vi "Complex Inverse Matrix.vi"(2 "matrix type":T1, 3 "Input Matrix":T2) -> (0 "error":i32, 1 "Inverse Matrix":T2)   [LabVIEW 2014, in "NI_AALBase.lvlib"]
doc: "Finds <B>Inverse Matrix</B>, if it exists, of <B>Input Matrix</B>. Wire data to the <B>Input Matrix</B> input to determine the polymorphic instance to use or manually select the instance."
uses:
  NI_AALBase.lvlib
  ComplexMatrix.ctl
  Matrix Type of Inverse Matrix.ctl
  NI_Matrix.lvlib
panel:
  # "Complex Inverse Matrix"
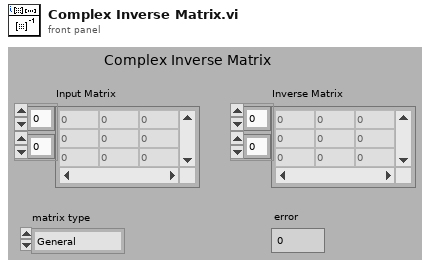
[diagram p1: front panel]
types:
  T1 = typedef "NI_AALBase.lvlib/Matrix Type of Inverse Matrix.ctl" = enum32{"General", "Positive Definite", "Lower Triangular", "Upper Triangular"}
  T2 = typedef "NI_Matrix.lvlib/ComplexMatrix.ctl" = cdb[][]
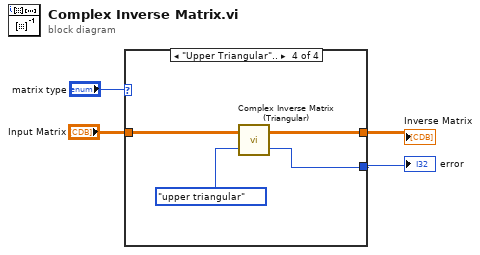
[diagram p0: block diagram]
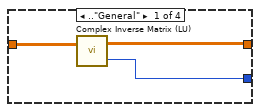
[diagram p2: hidden frame]
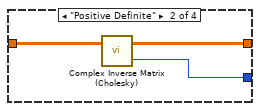
[diagram p3: hidden frame]
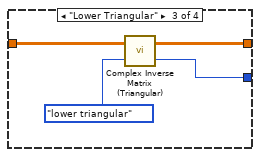
[diagram p4: hidden frame]
diagram:
  n1 = case shown="\"Upper Triangular\".." "matrix type" {
    tunnel: [w5 w9 w13 w17] -> w4
    tunnel: [w7 w10 w14 w18] -> w1
    tunnel: "Input Matrix" -> [w6 w8 w12 w16]
    frame .."General" {
      n2 = call "Complex Inverse Matrix (LU).vi"("A"=w6) -> ("error"=w5:i32, "Inverse Matrix"=w7:T2)  [unwired: 1 in]
    }
    frame "Positive Definite" {
      n3 = call "Complex Inverse Matrix (Cholesky).vi"("Input Matrix"=w8) -> ("error"=w9:i32, "Inverse Matrix"=w10:T2)  [unwired: 1 in]
    }
    frame "Lower Triangular" {
      n4 = call "Complex Inverse Matrix (Triangular).vi"("matrix type"=enum32{"lower triangular", "upper triangular"}."lower triangular", "A"=w12) -> ("error"=w13:i32, "Inverse Matrix"=w14:T2)
    }
    frame "Upper Triangular".. {
      n5 = call "Complex Inverse Matrix (Triangular).vi"("matrix type"=enum32{"lower triangular", "upper triangular"}."upper triangular", "A"=w16) -> ("error"=w17:i32, "Inverse Matrix"=w18:T2)
    }
  }
  "Inverse Matrix" <- w1
  "error" <- w4
